vi "init.vi"(8 "error in":errorcluster, 10 "module configuration":refnum<class "TBM module configuration.lvclass">, 11 "Simple Sequencer TBM runtime in":refnum<class "Simple Sequencer TBM runtime.lvclass">) -> (0 "error out":errorcluster, 1 "data allocations":T1, 2 "execution settings":T4, 3 "Simple Sequencer TBM runtime out":refnum<class "Simple Sequencer TBM runtime.lvclass">)   [LabVIEW 2014, in "Simple Sequencer TBM runtime.lvclass"]
doc: "Initializes the sequencer and all of the actions in the sequencer."
uses:
  Simple Sequencer TBM runtime.lvclass
  <vilib>/NI/Tag Bus Module Framework/runtime/execution settings.ctl
  <vilib>/NI/Tag Bus Module Framework/channel/data tables.ctl
  <vilib>/NI/Tag Bus/dictionary/data dictionary.lvclass
  <vilib>/NI/Tag Bus/dictionary table pair.ctl
  <vilib>/NI/Tag Bus/table/data table.ctl
  <vilib>/NI/Tag Bus Module Framework/module configuration/TBM module configuration.lvclass
  configuration/Simple Sequencer TBM configuration.lvclass
  sequencer states.ctl
  meta sequence definition.ctl
  configuration/Simple Sequencer TBM configuration.lvclass/Simple Sequencer TBM configuration.ctl
  sequence definition.ctl
  actions with configuration.ctl
  sequencer parent classes/action parent/action.lvclass
  <vilib>/NI/Tag Bus/table/transfer specification.ctl
  <vilib>/NI/Tag Bus/tag/Data Type.ctl
  Simple Sequencer TBM runtime.lvclass/Simple Sequencer TBM runtime.ctl
  configuration/Read sequencer name.vi
  configuration/Read shutdown action config.vi
  sequencer parent classes/action configuration parent/action configuration.lvclass
  <vilib>/NI/Tag Bus Module Framework/channel/TBM channel.lvclass
  <vilib>/NI/Tag Bus Module Framework/runtime/TBM module execution interface.lvclass
  <vilib>/NI/Tag Bus/table/data table.lvlib
  <vilib>/NI/Tag Bus/tag/tag descriptor.lvclass
  <vilib>/NI/Tag Bus/tag bus.lvlib
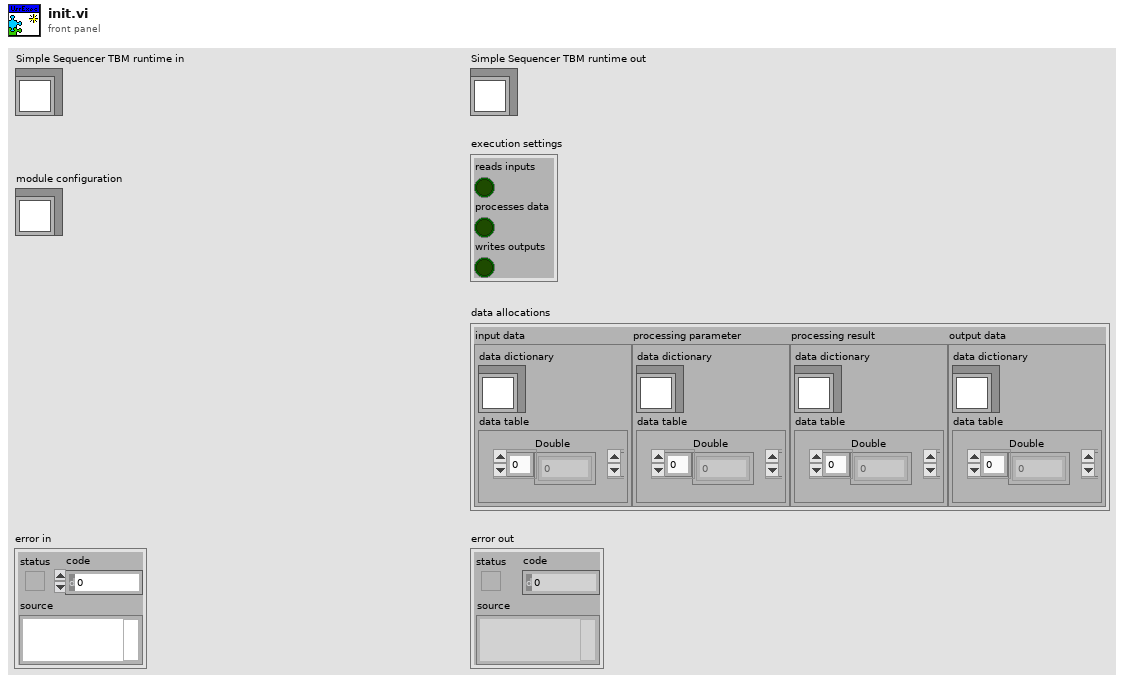
[diagram p1: front panel]
types:
  T1 = typedef "TBM channel.lvclass/data tables.ctl" = cluster{"input data":T2, "processing parameter":T2, "processing result":T2, "output data":T2}
  T2 = typedef "tag bus.lvlib/dictionary table pair.ctl" = cluster{"data dictionary":refnum<class "data dictionary.lvclass">, "data table":T3}
  T3 = typedef "tag bus.lvlib/data table.lvlib/data table.ctl" = cluster{"Double":dbl[], "Single":sgl[], "I64":i64[], "I32":i32[], "I16":i16[], "I8":i8[], "U64":u64[], "U32":u32[], "U16":u16[], "U8":u8[], "Boolean":bool[], "String":string[], "Array of Double":cluster{"DBL Array":dbl[]}[], "Array of Single":cluster{"SGL Array":sgl[]}[], "Array of I64":cluster{"I64 Array":i64[]}[], "Array of I32":cluster{"I32 Array":i32[]}[], "Array of I16":cluster{"I16 Array":i16[]}[], "Array of I8":cluster{"I8 Array":i8[]}[], "Array of U64":cluster{"U64 Array":u64[]}[], "Array of U32":cluster{"U32 Array":u32[]}[], "Array of U16":cluster{"U16 Array":u16[]}[], "Array of U8":cluster{"U8 Array":u8[]}[], "Array of Boolean":cluster{"Boolean Array":bool[]}[], "Array of String":cluster{"String Array":string[]}[]}
  T4 = typedef "TBM module execution interface.lvclass/execution settings.ctl" = cluster{"reads inputs":bool, "processes data":bool, "writes outputs":bool}
  T5 = typedef "Simple Sequencer TBM runtime.lvclass/meta sequence definition.ctl" = cluster{"sequence length":i32, "sequence pointers":i32[], "continue location":i32}
  T6 = typedef "Simple Sequencer TBM runtime.lvclass/sequencer states.ctl" = enum16{"stopped", "running", "paused"}
  T7 = typedef "Simple Sequencer TBM runtime.lvclass/sequence definition.ctl" = cluster{"sequence name":string, "sequence length":i32, "actions with configuration":T8[]}
  T8 = typedef "Simple Sequencer TBM runtime.lvclass/actions with configuration.ctl" = cluster{"action":refnum<class "action.lvclass">, "parameters":T3, "parameters specification":T9[], "results":T3, "results specification":T9[]}
  T9 = typedef "tag bus.lvlib/data table.lvlib/transfer specification.ctl" = cluster{"data type":T10, "sink indices":i32[], "source indices":i32[]}
  T10 = typedef "tag bus.lvlib/tag descriptor.lvclass/Data Type.ctl" = enum16{"Double", "Single", "I64", "I32", "I16", "I8", "U64", "U32", "U16", "U8", "Boolean", "String", "Array of Double", "Array of Single", "Array of I64", "Array of I32", "Array of I16", "Array of I8", "Array of U64", "Array of U32", "Array of U16", "Array of U8", "Array of Boolean", "Array of String"}
  T11 = typedef "Simple Sequencer TBM configuration.lvclass/sequence definition.ctl" = cluster{"sequence name":string, "action configs":refnum<class "action configuration.lvclass">[]}
  T12 = typedef "AMC.lvlib/Message Queue.ctl" = refnum<queue>
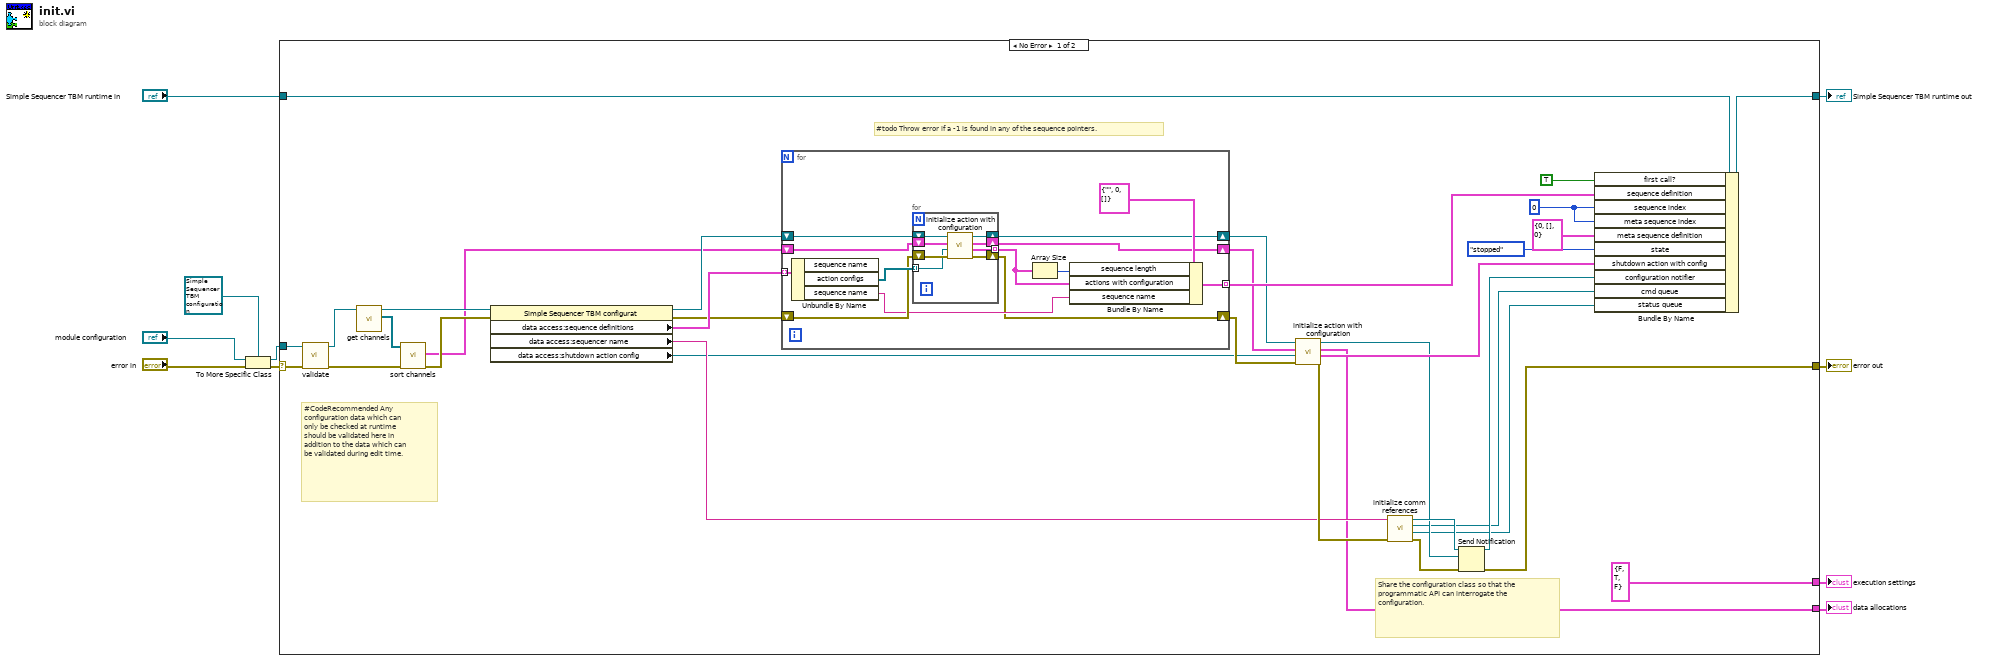
[diagram p0: block diagram]
diagram:
  n1 = To More Specific Class(target class=refnum<class "Simple Sequencer TBM configuration.lvclass"> refnum ("Synchronous module configuration"), reference="module configuration", error in="error in") -> (specific class reference=w9:refnum<class "Simple Sequencer TBM configuration.lvclass">, error out=w10:errorcluster)
  n2 = case shown="No Error" w10 {
    selector: w10 -> [w43 w66]
    tunnel: w9 -> [w42 _]
    tunnel: "Simple Sequencer TBM runtime in" -> [w39 w67]
    tunnel: [w38 w67] -> w5
    tunnel: [w24 w66] -> w4
    tunnel: [w12 _] -> w2
    tunnel: [T4 {"reads inputs"=FALSE, "processes data"=TRUE, "writes outputs"=FALSE} ("execution settings") _] -> w3
    frame No Error {
      w35 = 0 ("sequence index")
      # "Share the configuration class so that the programmatic API can interrogate the configuration."
      # "#todo Throw error if a -1 is found in any of the sequence pointers."
      # "#CodeRecommended Any configuration data which can only be checked at runtime should be validated here in addition to the data which can be validated during edit time."
      n3 = call-dynamic "validate.vi"("error in"=w43, "configuration in"=w42) -> ("error out"=w44:errorcluster, "configuration out"=w41:refnum<class "Simple Sequencer TBM configuration.lvclass">)  [unwired: 8 in]
      n4 = call-dynamic "get channels.vi"("Simple Sequencer TBM configuration in"=w41) -> ("channels"=w40:refnum<class "TBM channel.lvclass">[], "Simple Sequencer TBM configuration out"=w34:refnum<class "Simple Sequencer TBM configuration.lvclass">)  [unwired: 9 in]
      n5 = call <vilib>:"sort channels.vi"("error in"=w44, "channels in"=w40) -> ("error out"=w33:errorcluster, "data allocations"=w16:T1)  [unwired: 7 in, 1 out]
      n6 = property class="Simple Sequencer TBM configurat"(reference=w34, error in=w33) -> (reference out=w17:refnum<class "Simple Sequencer TBM configuration.lvclass">, error out=w18:errorcluster, "data access:sequence definitions"=w29:T11[], "data access:sequencer name"=w20:string, "data access:shutdown action config"=w11:refnum<class "action configuration.lvclass">)
      n7 = for {
        tunnel: w29 -> [w57] mode=indexing
        tunnel: [w55] -> w30 mode=indexing
        shift-right: [w48] -> w15
        shift-left: w16 -> [w50]
        shift-right: [w49] -> w14
        shift-left: w17 -> [w51]
        shift-right: [w45] -> w13
        shift-left: w18 -> [w52]
        n8 = Unbundle By Name(w57) -> ("action configs"=w53:refnum<class "action configuration.lvclass">[], "sequence name"=w47:string)  [unwired: 1 out]
        n9 = for {
          shift-right: [w65] -> w45
          shift-left: w52 -> [w64]
          tunnel: [w60] -> w46 mode=indexing
          shift-right: [w61] -> w49
          shift-left: w51 -> [w63]
          shift-right: [w59] -> w48
          shift-left: w50 -> [w62]
          tunnel: w53 -> [w58] mode=indexing
          n10 = call "initialize action with configuration.vi"("error in (no error)"=w64, "action configuration"=w58, "sequencer data allocations"=w62, "Simple Sequencer TBM configuration in"=w63) -> ("error out"=w65:errorcluster, "actions with configuration out"=w60:T8, "sequencer data allocations out"=w59:T1, "Simple Sequencer TBM configuration out"=w61:refnum<class "Simple Sequencer TBM configuration.lvclass">)  [unwired: 4 in]
        }
        n11 = Array Size(array=w46) -> (size(s)=w54:i32)
        n12 = Bundle By Name(cluster=T7 {"sequence name"="", "sequence length"=0, "actions with configuration"=[]}, "sequence length"=w54, "actions with configuration"=w46, "sequence name"=w47) -> (w55:T7)
      }
      n13 = call "initialize action with configuration.vi"("error in (no error)"=w13, "action configuration"=w11, "sequencer data allocations"=w15, "Simple Sequencer TBM configuration in"=w14) -> ("error out"=w25:errorcluster, "actions with configuration out"=w32:T8, "sequencer data allocations out"=w12:T1, "Simple Sequencer TBM configuration out"=w26:refnum<class "Simple Sequencer TBM configuration.lvclass">)  [unwired: 4 in]
      n14 = call "initialize comm references.vi"("error in (no error)"=w25, "sequencer name"=w20) -> ("error out"=w27:errorcluster, "message queue out"=w21:T12, "cmd queue out"=w22:T12, "config notifier out"=w28:refnum<notifier>)  [unwired: 6 in]
      n15 = Send Notification(notification=w26, notifier=w28, error in (no error)=w27) -> (notifier out=w23:refnum<notifier>, error out=w24:errorcluster)
      n16 = Bundle By Name(cluster=w39, "first call?"=TRUE, "sequence definition"=w30, "sequence index"=w35, "meta sequence index"=w35, "meta sequence definition"=T5 {"sequence length"=0, "sequence pointers"=[], "continue location"=0}, "state"=sequencer_states."stopped", "shutdown action with config"=w32, "configuration notifier"=w23, "cmd queue"=w22, "status queue"=w21) -> (w38:refnum<class "Simple Sequencer TBM runtime.lvclass">)
    }
    frame Error {
    }
  }
  "error out" <- w4
  "Simple Sequencer TBM runtime out" <- w5
  "execution settings" <- w3
  "data allocations" <- w2
